vi "Get States.vi"(8 "Error In":errorcluster, 11 "UIM In":refnum<data-value>) -> (0 "Error Out":errorcluster, 2 "States":string[](array[string]), 3 "UIM Out":refnum<data-value>)   [LabVIEW 2015, in "UIM.lvclass"]
doc: "List all the UI states currently stored and available in the UIM."
uses:
  UIM.lvclass
  UIM.lvclass/UIM.ctl
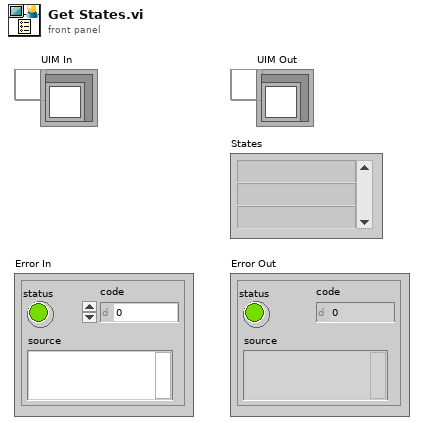
[diagram p1: front panel]
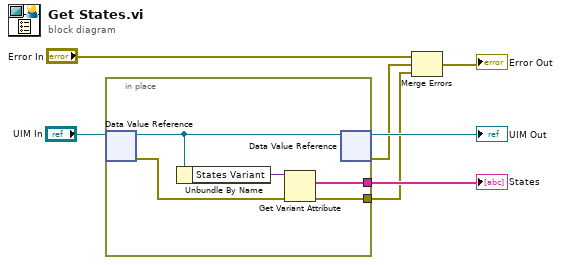
[diagram p0: block diagram]
diagram:
  n1 = in-place {
    in-place-border: [w9] -> w2
    in-place-border: [w10] -> w5
    n2 = in-place-dvr #1("UIM In") -> (w12:refnum<class "UIM.lvclass">, w8:errorcluster)
    n3 = Unbundle By Name(w12) -> ("States Variant"=w11:variant)
    n4 = Get Variant Attribute(Variant=w11, error in=w8) -> (names=w10:string[], error out=w9:errorcluster)  [unwired: 2 in, 2 out]
    n5 = in-place-dvr #1(w12) -> (→"UIM Out":refnum<data-value>, w1:errorcluster)
  }
  "States" <- w5
  n6 = Merge Errors("Error In", w1, w2) -> (→"Error Out":errorcluster)
